vi "H5Gget_info_by_name.vi"(3 "loc_id":i32, 4 "lapl_id":i32, 7 "group_name":string, 9 "error in (no error)":errorcluster) -> (0 "status":i32, 2 "group_info":T1 {"storage_type" items=["H5G_STORAGE_TYPE_UNKNOWN"=-1, "H5G_STORAGE_TYPE_SYMBOL_TABLE"=0, "H5G_STORAGE_TYPE_COMPACT"=1, "H5G_STORAGE_TYPE_DENSE"=2]}, 6 "error out":errorcluster)   [LabVIEW 2009]
uses:
  H5G_info_t.ctl
  H5G_storage_type_t.ctl
  hdf5dll.dll
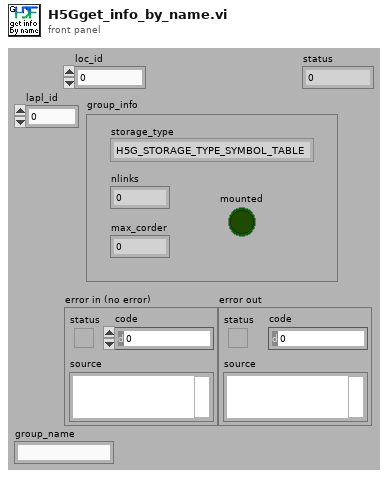
[diagram p1: front panel]
types:
  T1 = typedef "H5G_info_t.ctl" = cluster{"storage_type":T2, "nlinks":i64, "max_corder":i64, "mounted":bool}
  T2 = typedef "H5G_storage_type_t.ctl" = i32
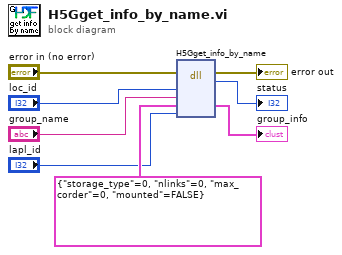
[diagram p0: block diagram]
diagram:
  n1 = dll-call lib="hdf5dll.dll" fn="H5Gget_info_by_name"(error in="error in (no error)", "loc_id"="loc_id", "group_name"="group_name", "group_info"=T1 {"storage_type"=0, "nlinks"=0, "max_corder"=0, "mounted"=FALSE} ("H5G_info_t"), "lapl_id"="lapl_id") -> (error out=→"error out":errorcluster, "return type"=→"status":i32, "group_info"=→"group_info":T1)  [unwired: 5 in, 1 out]
